vi "State Tracker for Debug.vi"(11 "State":string) -> ()   [LabVIEW 2012]
uses:
  <vilib>/Rock Robotics/WPI/DriverStation/DriverStationLCD/WPI_DriverStationLCDLCDLine.ctl
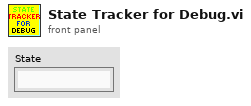
[diagram p1: front panel]
types:
  T1 = typedef "WPI_DriverStationLCDLCDLine.ctl" = enum16{"Main - Line 1", "User - Line 2", "User - Line 3", "User - Line 4", "User - Line 5", "User - Line 6"}
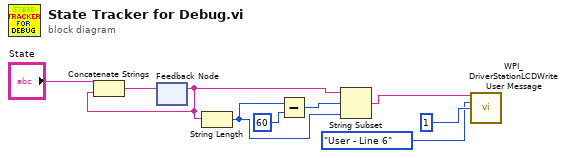
[diagram p0: block diagram]
diagram:
  n1 = feedback #1() -> (w5:string)  [unwired: 1 in]
  n2 = Concatenate Strings("State", w5) -> (w6:string)
  n3 = feedback-in #1(w6) -> ()
  n4 = String Length(string=w5) -> (length=w3:i32)
  n5 = Subtract(x=w3, y=60) -> (x-y=w2:i32)
  n6 = String Subset(string=w5, offset (0)=w2, length (rest)=w3) -> (substring=w1:string)
  n7 = call <vilib>:"WPI_DriverStationLCDWrite User Message.vi"("line text"=w1, "line"=WPI_DriverStationLCDLCDLine."User - Line 6", "starting column"=i8 1) -> ()  [unwired: 12 in, 1 out]
